vi "Fetch (Unscaled Int8).vi"(0 "VISA resource name":refnum<visa-resource-name>, 1 "Segment Index (0)":i32 format="%.0g", 5 "Measurement Source (1: Channel 1)":i32(ring)=1 items=["Channel 1"=1, "Channel 2"=2, "Channel 3"=3, "Channel 4"=4, "Function 1"=5, "Function 2"=6, "Function 3"=7, "Function 4"=8, "Memory 1"=9, "Memory 2"=10, "Memory 3"=11, "Memory 4"=12], 7 "Number of Samples (1000)":i32=10000 caption="Number of Samples (10000)", 9 "Maximum Time (10000ms)":u32=10000, 11 "error in (no error)":errorcluster, 12 "Offset (0)":i32) -> (4 "VISA resource name out":refnum<visa-resource-name>, 6 "Waveform Information":T1, 8 "Waveform Data":i8[](array[numeric]), 15 "error out":errorcluster)   [LabVIEW 2020, in "Agilent 90000 Series.lvlib"]
doc: "Fetches the unscaled raw byte data from instrument. Use this VI under byte data format configuration."
uses:
  Agilent 90000 Series.lvlib
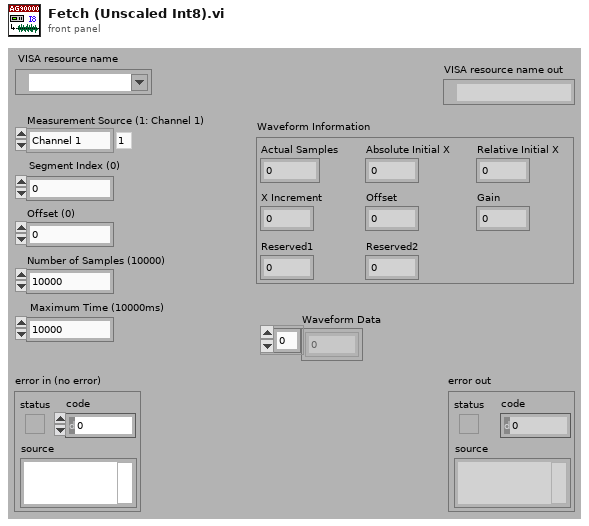
[diagram p1: front panel]
types:
  T1 = cluster{"Actual Samples":i32, "Absolute Initial X":dbl, "Relative Initial X":dbl, "X Increment":dbl, "Offset":dbl, "Gain":dbl, "Reserved1":dbl, "Reserved2":dbl}
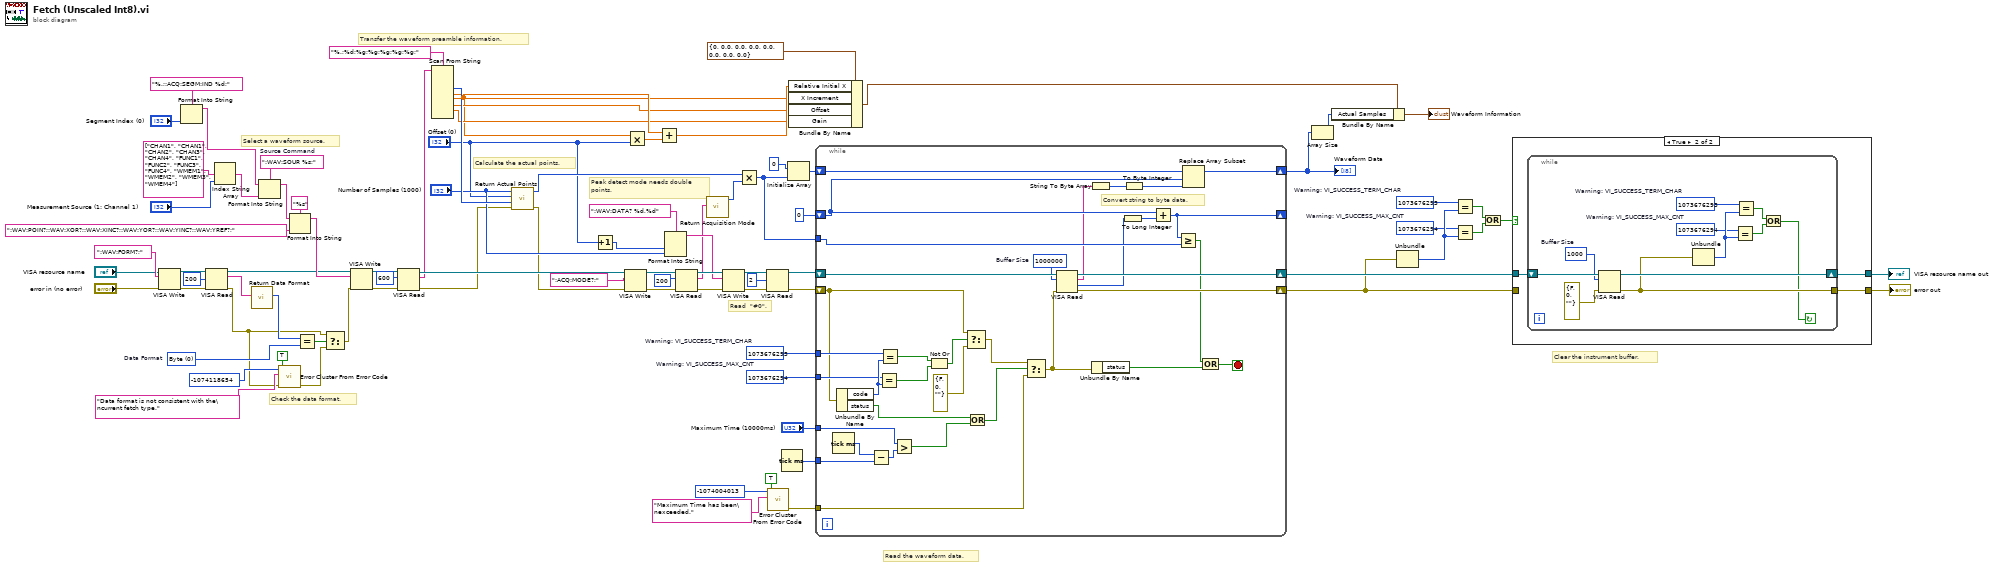
[diagram p0: block diagram]
diagram:
  w28 = u16 0 items=["Byte", "Word", "Others"]  # Data Format
  w73 = 1073676294  # Warning: VI_SUCCESS_MAX_CNT
  w72 = 1073676293  # Warning: VI_SUCCESS_TERM_CHAR
  w65 = 1073676294  # Warning: VI_SUCCESS_MAX_CNT
  w64 = 1073676293  # Warning: VI_SUCCESS_TERM_CHAR
  w86 = ":WAV:SOUR %s;"  # Source Command
  # "Check the data format."
  # "Peak detect mode needs double\npoints."
  # "Calculate the actual points."
  # "Read  \"#0\"."
  # "Clear the instrument buffer."
  # "Read the waveform data."
  # "Select a waveform source."
  # "Transfer the waveform preamble information."
  n1 = VISA Write(VISA resource name="VISA resource name", write buffer=":WAV:FORM?;", error in (no error)="error in (no error)") -> (VISA resource name out=w23:refnum<visa-resource-name>, error out=w24:errorcluster)  [unwired: 1 out]
  n2 = Format Into String(format string="%.;:ACQ:SEGM:IND %d;", "Segment Index (0)") -> (resulting string=w2:string)  [unwired: 2 in, 1 out]
  n3 = VISA Read(VISA resource name=w23, byte count=u32 200, error in (no error)=w24) -> (VISA resource name out=w22:refnum<visa-resource-name>, read buffer=w20:string, error out=w5:errorcluster)  [unwired: 1 out]
  n4 = Index String Array(1:"Measurement Source (1: Channel 1)", 2:string[] ["CHAN1", "CHAN1", "CHAN2", "CHAN3", "CHAN4", "FUNC1", "FUNC2", "FUNC3", "FUNC4", "WMEM1", "WMEM2", "WMEM3", "WMEM4"] ("subarray 2")) -> (0:w81:string)  [unwired: 1 out]
  n5 = call "Return Data Format.vi"("String In"=w20) -> ("Data Format"=w34:u16)  [unwired: 1 in, 9 out]
  n6 = Format Into String(format string=w86, initial string=w2, w81) -> (resulting string=w84:string)  [unwired: 1 in, 1 out]
  n7 = call <vilib>:"Error Cluster From Error Code.vi"("show call chain? (False)"=TRUE, "error in (no error)"=w5, "error message (\"\")"="Data format is not consistent with the\ncurrent fetch type." ("error message (\"\")"), "error code (0)"=-1074118654) -> ("error out"=w29:errorcluster)  [unwired: 5 out]
  n8 = Format Into String(format string="%s", initial string=w84, ":WAV:POIN?;:WAV:XOR?;:WAV:XINC?;:WAV:YOR?;:WAV:YINC?;:WAV:YREF?;" ("X/Y Increment, Origin, and Offset")) -> (resulting string=w83:string)  [unwired: 1 in, 1 out]
  n9 = Equal?(x=w34, y=w28) -> (x = y?=w33:bool)
  n10 = Select(t=w5, s=w33, f=w29) -> (s? t:f=w19:errorcluster)
  n11 = VISA Write(VISA resource name=w22, write buffer=w83, error in (no error)=w19) -> (VISA resource name out=w89:refnum<visa-resource-name>, error out=w88:errorcluster)  [unwired: 1 out]
  n12 = VISA Read(VISA resource name=w89, byte count=u32 600, error in (no error)=w88) -> (VISA resource name out=w56:refnum<visa-resource-name>, read buffer=w43:string, error out=w7:errorcluster)  [unwired: 1 out]
  n13 = Scan From String(format string="%.;%d;%g;%g;%g;%g;%g;", input string=w43) -> (output 1=w44:i32, output 2=w42:dbl, output 3=w10:dbl, output 4=w15:dbl, output 5=w14:dbl)  [unwired: 2 in, 10 out]
  n14 = call "Return Actual Points.vi"("error in (no error)"=w7, "Total Points (2000)"=w44, "Offset (0)"="Offset (0)", "Number of Samples (1000)"="Number of Samples (1000)") -> ("error out"=w6:errorcluster, "Actual Points"=w39:i32)  [unwired: 6 out]
  n15 = Increment(x="Offset (0)") -> (x+1=w11:i32)
  n16 = VISA Write(VISA resource name=w56, write buffer=":ACQ:MODE?;", error in (no error)=w6) -> (VISA resource name out=w55:refnum<visa-resource-name>, error out=w54:errorcluster)  [unwired: 1 out]
  n17 = Multiply(x=w10, y="Offset (0)") -> (x*y=w48:dbl)
  n18 = Add(x=w42, y=w48) -> (x+y=w47:dbl)
  n19 = Format Into String(format string=":WAV:DATA? %d,%d", w11, "Number of Samples (1000)") -> (resulting string=w49:string)  [unwired: 2 in, 1 out]
  n20 = VISA Read(VISA resource name=w55, byte count=u32 200, error in (no error)=w54) -> (VISA resource name out=w53:refnum<visa-resource-name>, read buffer=w12:string, error out=w8:errorcluster)  [unwired: 1 out]
  n21 = call "Return Acquisition Mode.vi"("Acquisition Mode"=w12) -> ("Multiply Factor"=w13:i32)  [unwired: 10 out]
  n22 = VISA Write(VISA resource name=w53, write buffer=w49, error in (no error)=w8) -> (VISA resource name out=w59:refnum<visa-resource-name>, error out=w58:errorcluster)  [unwired: 1 out]
  n23 = Multiply(x=w39, y=w13) -> (x*y=w38:i32)
  n24 = VISA Read(VISA resource name=w59, byte count=u32 2, error in (no error)=w58) -> (VISA resource name out=w40:refnum<visa-resource-name>, error out=w41:errorcluster)  [unwired: 2 out]
  n25 = call <vilib>:"Error Cluster From Error Code.vi"("show call chain? (False)"=TRUE, "error message (\"\")"="Maximum Time has been\nexceeded." ("error message (\"\")"), "error code (0)"=-1074004013) -> ("error out"=w71:errorcluster)  [unwired: 1 in, 5 out]
  n26 = Tick Count (ms)() -> (millisecond timer value=w70:u32)
  n27 = Initialize Array(i8 0 ("element"), w38) -> (w62:i8[])
  n28 = Bundle By Name(cluster=T1 {"Actual Samples"=0, "Absolute Initial X"=0.0, "Relative Initial X"=0.0, "X Increment"=0.0, "Offset"=0.0, "Gain"=0.0, "Reserved1"=0.0, "Reserved2"=0.0} ("Waveform Information 2"), "Relative Initial X"=w47, "X Increment"=w10, "Offset"=w15, "Gain"=w14) -> (w46:T1)
  n29 = while {
    shift-right: [w119] -> w78
    shift-left: w41 -> [w107]
    shift-right: [w124] -> w79
    shift-left: w40 -> [w123]
    shift-right: [w120] -> w1
    shift-left: w62 -> [w121]
    tunnel: w38 -> [w116]
    tunnel: w64 -> [w109]
    tunnel: w65 -> [w108]
    tunnel: "Maximum Time (10000ms)" -> [w104]
    tunnel: w70 -> [w103]
    tunnel: w71 -> [w98]
    shift-right: [w117] -> _
    shift-left: 0 ("index") -> [w118]
    stop <- w95 stop-if-true
    w122 = u32 1000000  # Buffer Size
    # "Convert string to byte data."
    n30 = Tick Count (ms)() -> (millisecond timer value=w105:u32)
    n31 = Unbundle By Name(w107) -> ("code"=w110:i32, "status"=w102:bool)
    n32 = Subtract(x=w105, y=w103) -> (x-y=w106:u32)
    n33 = Equal?(x=w108, y=w110) -> (x = y?=w113:bool)
    n34 = Equal?(x=w109, y=w110) -> (x = y?=w114:bool)
    n35 = Greater?(x=w104, y=w106) -> (0:w101:bool)
    n36 = Not Or(1:w113, 2:w114) -> (0:w112:bool)
    n37 = Select(t=w107, s=w112, f=errorcluster {"status"=FALSE, "code"=0, "source"=""} ("error in (no error)")) -> (s? t:f=w100:errorcluster)
    n38 = Or(x=w102, y=w101) -> (x .or. y?=w99:bool)
    n39 = Select(t=w100, s=w99, f=w98) -> (s? t:f=w97:errorcluster)
    n40 = VISA Read(VISA resource name=w123, byte count=w122, error in (no error)=w97) -> (VISA resource name out=w124:refnum<visa-resource-name>, read buffer=w93:string, return count=w94:u32, error out=w119:errorcluster)
    n41 = String To Byte Array(string=w93) -> (unsigned byte array=w92:u8[])
    n42 = Unbundle By Name(w97) -> ("status"=w96:bool)
    n43 = To Long Integer(number=w94) -> (32bit integer=w90:i32)
    n44 = To Byte Integer(number=w92) -> (8bit integer=w91:i8[])
    n45 = Add(x=w118, y=w90) -> (x+y=w117:i32)
    n46 = Greater Or Equal?(x=w117, y=w116) -> (x >= y?=w115:bool)
    n47 = Replace Array Subset(array=w121, new element=w91, index=w118) -> (w120:i8[])
    n48 = Compound Arithmetic op=OR(w115, w96) -> (w95:bool)
  }
  "Waveform Data" <- w1
  n49 = Array Size(array=w1) -> (size(s)=w16:i32)
  n50 = Bundle By Name(cluster=w46, "Actual Samples"=w16) -> (→"Waveform Information":T1)
  n51 = Unbundle(w78) -> ("code"=w74:i32)  [unwired: 2 out]
  n52 = Equal?(x=w73, y=w74) -> (x = y?=w76:bool)
  n53 = Equal?(x=w72, y=w74) -> (x = y?=w77:bool)
  n54 = Or(x=w77, y=w76) -> (x .or. y?=w75:bool)
  n55 = case shown="True" w75 {
    tunnel: w79 -> [w126 w129]
    tunnel: w78 -> [w125 _]
    tunnel: [w126 w128] -> w36
    tunnel: [w125 w127] -> w35
    frame False {
    }
    frame True {
      n56 = while {
        shift-right: [w139] -> w128
        shift-left: w129 -> [w140]
        tunnel: [w132] -> w127
        stop <- w131 continue-if-true
        w134 = 1073676294  # Warning: VI_SUCCESS_MAX_CNT
        w133 = 1073676293  # Warning: VI_SUCCESS_TERM_CHAR
        w138 = u32 1000  # Buffer Size
        n57 = VISA Read(VISA resource name=w140, byte count=w138, error in (no error)=errorcluster {"status"=FALSE, "code"=0, "source"=""}) -> (VISA resource name out=w139:refnum<visa-resource-name>, error out=w132:errorcluster)  [unwired: 2 out]
        n58 = Unbundle(w132) -> ("code"=w135:i32)  [unwired: 2 out]
        n59 = Equal?(x=w134, y=w135) -> (x = y?=w136:bool)
        n60 = Equal?(x=w133, y=w135) -> (x = y?=w137:bool)
        n61 = Or(x=w137, y=w136) -> (x .or. y?=w131:bool)
      }
    }
  }
  "error out" <- w35
  "VISA resource name out" <- w36
